vi "scan test.vi"() -> ()   [LabVIEW 2013]
uses:
  Program Files/National Instruments/LabVIEW 2013/examples/Instrument IO/Serial/support/Serial - Settings.ctl
  <vilib>/Instr/_visa.llb/VISA Configure Serial Port (Instr).vi
panel:
  in  "VISA resource name 2":refnum<visa-resource-name>="COM1"
  out "Response 2":string
  out "bytes read 2":u32
  in  "Boolean 2":bool
  in  "Boolean":bool
  in  "Serial Settings":T1={"baud rate"=57600, "data bits"=8, "parity"=enum."None", "stop bits"=10, "flow control"=0} {"flow control" items=["None"=0, "XON/XOFF"=1, "RTS/CTS"=2, "DTR/DSR"=4]; "stop bits" items=["1.0"=10, "1.5"=15, "2.0"=20]; "data bits" min=5 max=8 step=1; "baud rate" items=["75"=75, "110"=110, "134"=134, "150"=150, "300"=300, "600"=600, "1200"=1200, "1800"=1800, "2400"=2400, "4800"=4800, "7200"=7200, "9600"=9600, "14400"=14400, "19200"=19200, "28800"=28800, "38400"=38400, "56000"=56000, "57600"=57600, "115200"=115200, "128000"=128000, "230400"=230400]}
  out "bytes read":u32
  out "Response":string
  in  "delay before read (ms)":u32=500
  in  "VISA resource name":refnum<visa-resource-name>="COM1"
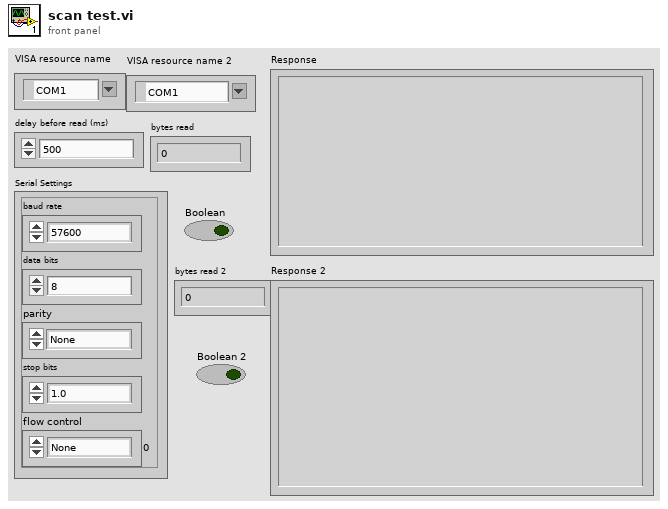
[diagram p1: front panel]
types:
  T1 = typedef "Serial - Settings.ctl" = cluster{"baud rate":u32, "data bits":u16, "parity":enum16{"None", "Odd", "Even", "Mark", "Space"}, "stop bits":u16, "flow control":u16}
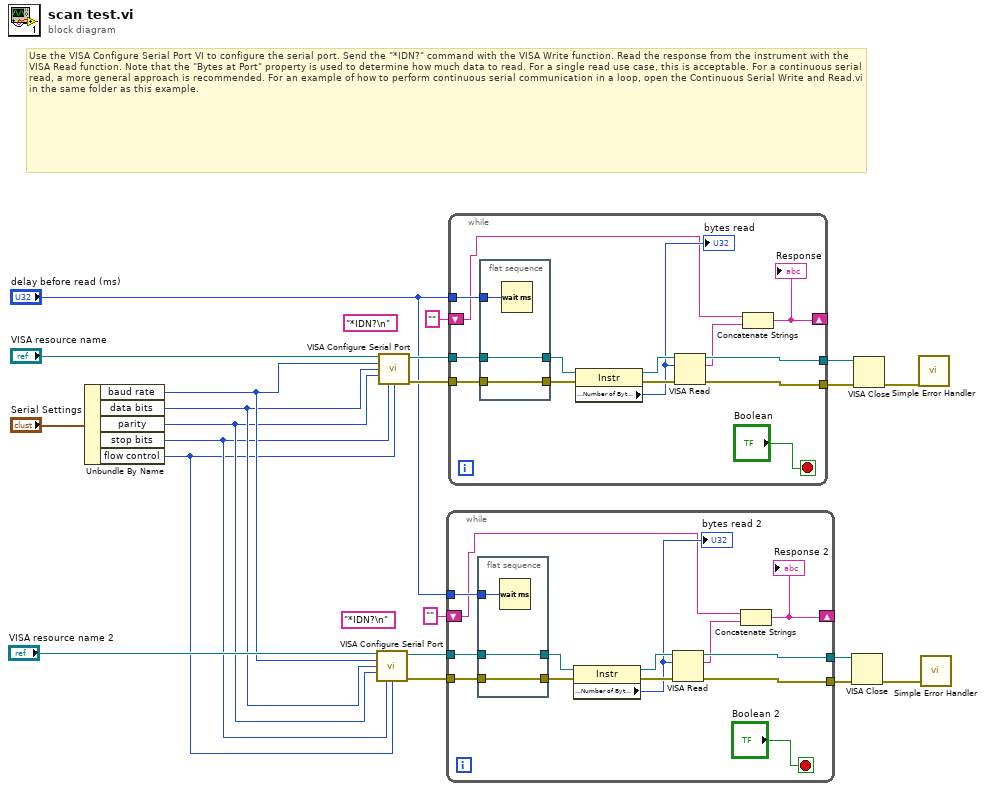
[diagram p0: block diagram]
diagram:
  (unwired) "*IDN?\n" ("Command")
  (unwired) "*IDN?\n" ("Command")
  # "Use the VISA Configure Serial Port VI to configure the serial port. Send the \"*IDN?\" command with the VISA Write function. Read the response from the instrument with the VISA Read function. Note that the \"Bytes at Port\" property is used to determine how much data to read. For a single read use case, this is acceptable. For a continuous serial read, a more general approach is recommended. For an example of how to perform continuous serial communication in a loop, open the Continuous Serial Write and Read.vi in the same folder as this example."
  n1 = Unbundle By Name("Serial Settings") -> ("baud rate"=w7:u32, "data bits"=w6:u16, "parity"=w5:enum16{"None", "Odd", "Even", "Mark", "Space"}, "stop bits"=w4:u16, "flow control"=w3:u16)
  n2 = call-poly "VISA Configure Serial Port"("VISA resource name"="VISA resource name 2", "baud rate (9600)"=w7, "data bits (8)"=w6, "parity (0:none)"=w5, "stop bits (10: 1 bit)"=w4, "flow control (0:none)"=w3) -> ("VISA resource name out"=w11:refnum<visa-resource-name>, "error out"=w12:errorcluster)  [unwired: 3 in, 5 out]
  n3 = call-poly "VISA Configure Serial Port"("VISA resource name"="VISA resource name", "baud rate (9600)"=w7, "data bits (8)"=w6, "parity (0:none)"=w5, "stop bits (10: 1 bit)"=w4, "flow control (0:none)"=w3) -> ("VISA resource name out"=w16:refnum<visa-resource-name>, "error out"=w15:errorcluster)  [unwired: 3 in, 5 out]
  n4 = while {
    tunnel: [w35] -> w9
    tunnel: [w34] -> w10
    tunnel: "delay before read (ms)" -> [w31]
    tunnel: w11 -> [w27]
    tunnel: w12 -> [w26]
    shift-right: [w23] -> _
    shift-left: "" -> [w24]
    stop <- "Boolean 2" stop-if-true
    n5 = flat-sequence {
      tunnel: w26 -> [w37]
      tunnel: [w37] -> w33
      tunnel: w27 -> [w36]
      tunnel: [w36] -> w32
      tunnel: w31 -> [w38]
      frame #0 {
        n6 = Wait (ms)(milliseconds to wait=w38) -> ()  [unwired: 1 out]
      }
    }
    n7 = property class="Instr"(reference=w32, error in=w33) -> (reference out=w30:refnum<visa-resource-name>, error out=w29:errorcluster, "Serial Settings:Number of Bytes at Serial Port"=w28:u32)
    "bytes read 2" <- w28
    n8 = VISA Read(VISA resource name=w30, byte count=w28, error in (no error)=w29) -> (VISA resource name out=w34:refnum<visa-resource-name>, read buffer=w25:string, error out=w35:errorcluster)  [unwired: 1 out]
    n9 = Concatenate Strings(w24, w25) -> (w23:string)
    "Response 2" <- w23
  }
  n10 = while {
    tunnel: [w52] -> w20
    tunnel: [w51] -> w19
    tunnel: "delay before read (ms)" -> [w48]
    tunnel: w16 -> [w44]
    tunnel: w15 -> [w43]
    shift-right: [w40] -> _
    shift-left: "" -> [w41]
    stop <- "Boolean" stop-if-true
    n11 = flat-sequence {
      tunnel: w43 -> [w54]
      tunnel: [w54] -> w50
      tunnel: w44 -> [w53]
      tunnel: [w53] -> w49
      tunnel: w48 -> [w55]
      frame #0 {
        n12 = Wait (ms)(milliseconds to wait=w55) -> ()  [unwired: 1 out]
      }
    }
    n13 = property class="Instr"(reference=w49, error in=w50) -> (reference out=w47:refnum<visa-resource-name>, error out=w46:errorcluster, "Serial Settings:Number of Bytes at Serial Port"=w45:u32)
    "bytes read" <- w45
    n14 = VISA Read(VISA resource name=w47, byte count=w45, error in (no error)=w46) -> (VISA resource name out=w51:refnum<visa-resource-name>, read buffer=w42:string, error out=w52:errorcluster)  [unwired: 1 out]
    n15 = Concatenate Strings(w41, w42) -> (w40:string)
    "Response" <- w40
  }
  n16 = VISA Close(VISA resource name=w10, error in (no error)=w9) -> (error out=w2:errorcluster)
  n17 = VISA Close(VISA resource name=w19, error in (no error)=w20) -> (error out=w18:errorcluster)
  n18 = call <vilib>:"Simple Error Handler.vi"("error in (no error)"=w18) -> ()  [unwired: 1 in, 8 out]
  n19 = call <vilib>:"Simple Error Handler.vi"("error in (no error)"=w2) -> ()  [unwired: 1 in, 8 out]
